vi "MU Save Params.vi"(8 "error in (no error)":errorcluster, 10 "filepath":string, 11 "handle":u64) -> (0 "error out (no error)":errorcluster, 3 "function return":u32)   [LabVIEW 2017, in "MU_3SL_interface.lvlib"]
uses:
  MU_3SL_interface.lvlib
  lib/MU_3SL_interface.dll
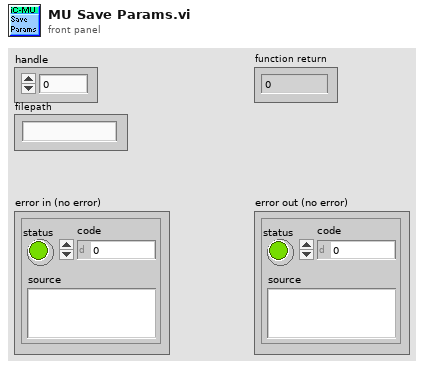
[diagram p1: front panel]
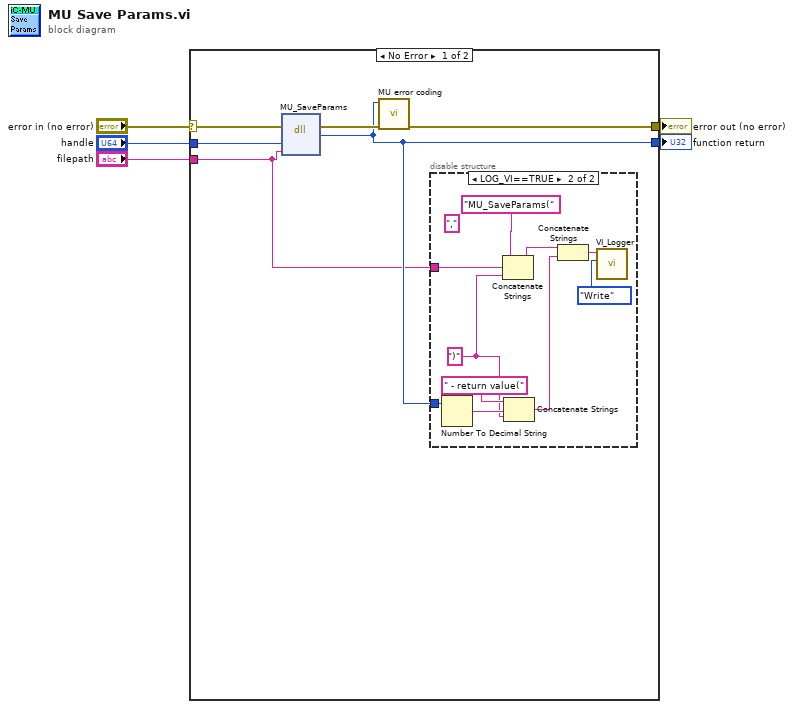
[diagram p0: block diagram]
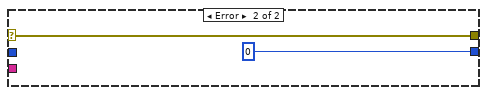
[diagram p3: hidden frame]
diagram:
  n1 = case shown="No Error" "error in (no error)" {
    selector: "error in (no error)" -> [w8 w23]
    tunnel: [w7 u32 0] -> w5
    tunnel: "handle" -> [w11 _]
    tunnel: "filepath" -> [w6 _]
    tunnel: [w9 w23] -> w2
    frame No Error {
      n2 = dll-call lib="C:/Users/bes/AppData/Roaming/work/mu_9so/icsubmodules/soft_mu_3sl_master/lv_interface/lib/MU_3SL_interface**.*" fn="MU_SaveParams"(error in=w8, "handle"=w11, "filepath"=w6) -> (error out=w10:errorcluster, "return type"=w7:u32)  [unwired: 4 in, 1 out]
      n3 = call "MU error coding.vi"("error in (no error)"=w10, "function return in"=w7) -> ("error out"=w9:errorcluster)  [unwired: 9 in]
      n4 = disable-structure shown="LOG_VI==TRUE" {
        disable-tunnel: w7 -> [_ w19]
        disable-tunnel: w6 -> [_ w13]
        frame condition #0 {
        }
        frame condition #1 (active) {
          w12 = ")" ("string")
          (unwired) "," ("string")
          n5 = Number To Decimal String(number=w19) -> (decimal integer string=w18:string)  [unwired: 1 in]
          n6 = Concatenate Strings("MU_SaveParams(" ("Info in"), w13, w12) -> (w17:string)
          n7 = Concatenate Strings(" - return value(" ("string"), w18, w12) -> (w16:string)
          n8 = Concatenate Strings(w17, w16) -> (w15:string)
          n9 = call "VI_Logger.vi"("Action (Read)"=enum16{"Write", "Read"}."Write", "Info in"=w15) -> ()  [unwired: 8 in, 2 out]
        }
      }
    }
    frame Error {
    }
  }
  "function return" <- w5
  "error out (no error)" <- w2
